vi "Write Websocket Server Message Transport.vi"(10 "Stream Mediator.lvlib:Message Transport Interface.lvclass":refnum<class "Message Transport Interface.lvclass">, 11 "Websocket Message Broker Interface Ref in":refnum<class "Websocket Message Broker Interface Ref.lvclass">) -> (3 "Websocket Message Broker Interface Ref out":refnum<class "Websocket Message Broker Interface Ref.lvclass">)   [LabVIEW 2016, in "Stream Mediator.lvlib" / "Websocket Message Broker Interface Ref.lvclass"]
uses:
  <userlib>/Composed Systems/Stream/Mediator/Classes/Websocket Message Broker Interface Ref/Websocket Message Broker Interface Ref.lvclass
  <userlib>/Composed Systems/Stream/Mediator/Classes/Message Transport Interface/Message Transport Interface.lvclass
  <userlib>/Composed Systems/Stream/Mediator/Classes/Websocket Message Broker Interface Ref/Websocket Message Broker Interface Ref.lvclass/Websocket Message Broker Interface Ref.ctl
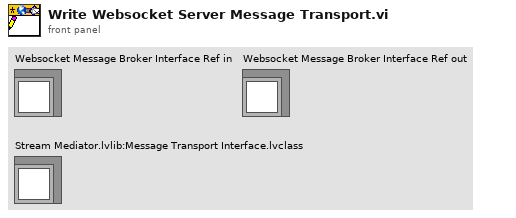
[diagram p1: front panel]
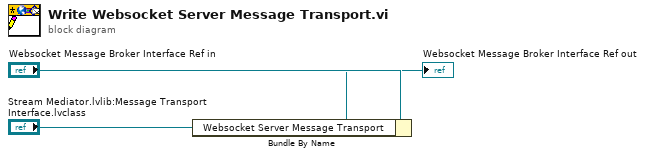
[diagram p0: block diagram]
diagram:
  n1 = Bundle By Name(cluster="Websocket Message Broker Interface Ref in", "Websocket Server Message Transport"="Stream Mediator.lvlib:Message Transport Interface.lvclass") -> (→"Websocket Message Broker Interface Ref out":refnum<class "Websocket Message Broker Interface Ref.lvclass">)
